vi "Class Data has DVR.vi"(10 "Ref Data Ctl":refnum<vi>, 11 "Class Data":refnum<vi>) -> (3 "Has DVR?":bool)   [LabVIEW 2018, in "LVClassByRef.lvlib"]
uses:
  <resource>/Framework/Providers/LVClassByRef/LVClassByRef.lvlib
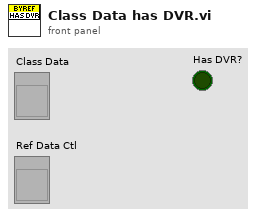
[diagram p1: front panel]
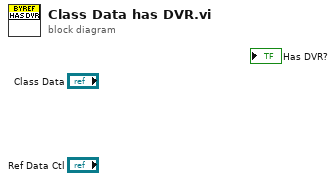
[diagram p0: block diagram]
diagram:
